vi "RichToFlatAcquisition_Control_Stream.vi"(5 "OutputClusterType":T1, 11 "InputCluster":T2) -> (3 "OutputCluster":T1)   [LabVIEW 2021, in "Stream_server.lvlib"]
uses:
  Stream_server.lvlib
  Acquisition_Control_Stream.ctl
  Acquisition_Control_Stream_Flat.ctl
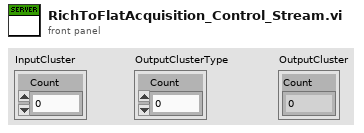
[diagram p1: front panel]
types:
  T1 = typedef "Stream_server.lvlib/Acquisition_Control_Stream_Flat.ctl" = cluster{"Count":i32}
  T2 = typedef "Stream_server.lvlib/Acquisition_Control_Stream.ctl" = cluster{"Count":i32}
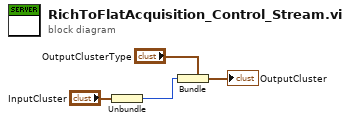
[diagram p0: block diagram]
diagram:
  n1 = Unbundle "Unbundle"("InputCluster") -> ("Count"=w1:i32)
  n2 = Bundle "Bundle"(cluster="OutputClusterType", "Count"=w1) -> (→"OutputCluster":T1)
